vi "Global graph.vi"() -> ()   [LabVIEW 2012]
uses:
  Graph.ctl
panel:
  out "Dust Distribution":T1
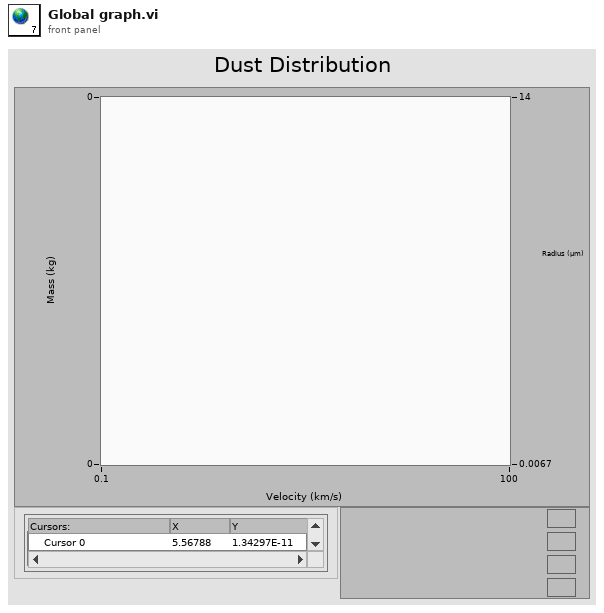
[diagram p1: front panel]
types:
  T1 = typedef "Graph.ctl" = cluster{cluster{"Vnoise":dbl, "Vnoise":dbl}[]}[]
diagram:
